vi "Convert64PinPGAToInputs.vi"(11 "64-Pin PGA":T2) -> (3 "Inputs":T1[](array[typedef]))   [LabVIEW 2012, in "Virtual-PGA.lvlib"]
uses:
  Virtual-PGA.lvlib
  Public/Controls/64PinPGAPattern.ctl
  Public/Controls/64PinPGAPads1-16.ctl
  Public/Controls/64PinPGAPad1-16.ctl
  Public/Controls/64PinPGAPads17-32.ctl
  Public/Controls/64PinPGAPad17-32.ctl
  Public/Controls/64PinPGAPads33-48.ctl
  Public/Controls/64PinPGAPad33-48.ctl
  Public/Controls/64PinPGAPads49-64.ctl
  Public/Controls/64PinPGAPad49-64.ctl
  Public/Controls/Input.ctl
panel:
  # "Name:"
  # "Inputs:"
  # "Description:"
  # "Y4:"
  # "Y3:"
  # "Y2:"
  # "Y1:"
  # "49"
  # "50"
  # "51"
  # "52"
  # "53"
  # "54"
  # "55"
  # "56"
  # "57"
  # "58"
  # "59"
  # "60"
  # "61"
  # "62"
  # "63"
  # "64"
  # "1"
  # "2"
  # "3"
  # "4"
  # "5"
  # "6"
  # "7"
  # "8"
  # "9"
  # "10"
  # "11"
  # "12"
  # "13"
  # "14"
  # "15"
  # "16"
  # "32"
  # "31"
  # "30"
  # "29"
  # "28"
  # "27"
  # "26"
  # "25"
  # "24"
  # "23"
  # "22"
  # "21"
  # "20"
  # "19"
  # "18"
  # "17"
  # "48"
  # "47"
  # "46"
  # "45"
  # "44"
  # "43"
  # "42"
  # "41"
  # "40"
  # "39"
  # "38"
  # "37"
  # "36"
  # "35"
  # "34"
  # "33"
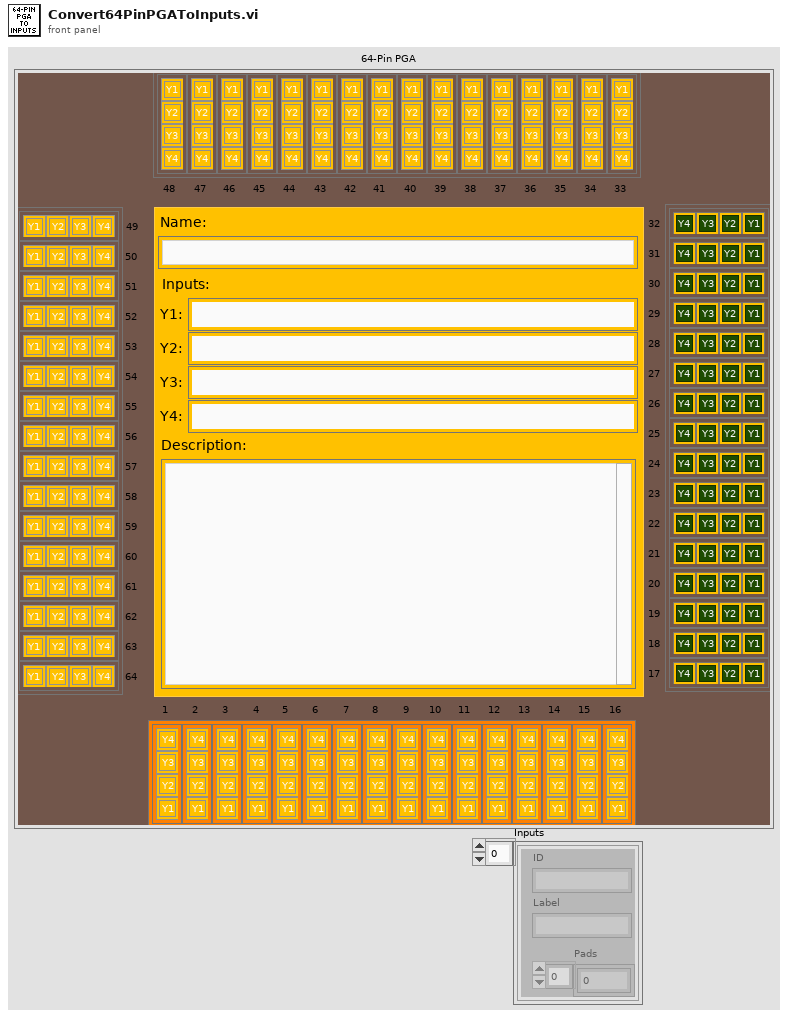
[diagram p1: front panel]
types:
  T1 = typedef "Virtual-PGA.lvlib/Input.ctl" = cluster{"ID":string, "Label":string, "Pads":u32[]}
  T2 = typedef "Virtual-PGA.lvlib/64PinPGAPattern.ctl" = cluster{"Name":string, "Description":string, "Y1 Label":string, "Y2 Label":string, "Y3 Label":string, "Y4 Label":string, "Pads 1-16":T3, "Pads 17-32":T5, "Pads 33-48":T7, "Pads 49-64":T9}
  T3 = typedef "Virtual-PGA.lvlib/64PinPGAPads1-16.ctl" = T4[]
  T4 = typedef "Virtual-PGA.lvlib/64PinPGAPad1-16.ctl" = cluster{"Y1":bool, "Y2":bool, "Y3":bool, "Y4":bool}
  T5 = typedef "Virtual-PGA.lvlib/64PinPGAPads17-32.ctl" = T6[]
  T6 = typedef "Virtual-PGA.lvlib/64PinPGAPad17-32.ctl" = cluster{"Y1":bool, "Y2":bool, "Y3":bool, "Y4":bool}
  T7 = typedef "Virtual-PGA.lvlib/64PinPGAPads33-48.ctl" = T8[]
  T8 = typedef "Virtual-PGA.lvlib/64PinPGAPad33-48.ctl" = cluster{"Y1":bool, "Y2":bool, "Y3":bool, "Y4":bool}
  T9 = typedef "Virtual-PGA.lvlib/64PinPGAPads49-64.ctl" = T10[]
  T10 = typedef "Virtual-PGA.lvlib/64PinPGAPad49-64.ctl" = cluster{"Y1":bool, "Y2":bool, "Y3":bool, "Y4":bool}
  T11 = cluster{"Y1":bool, "Y2":bool, "Y3":bool, "Y4":bool}[]
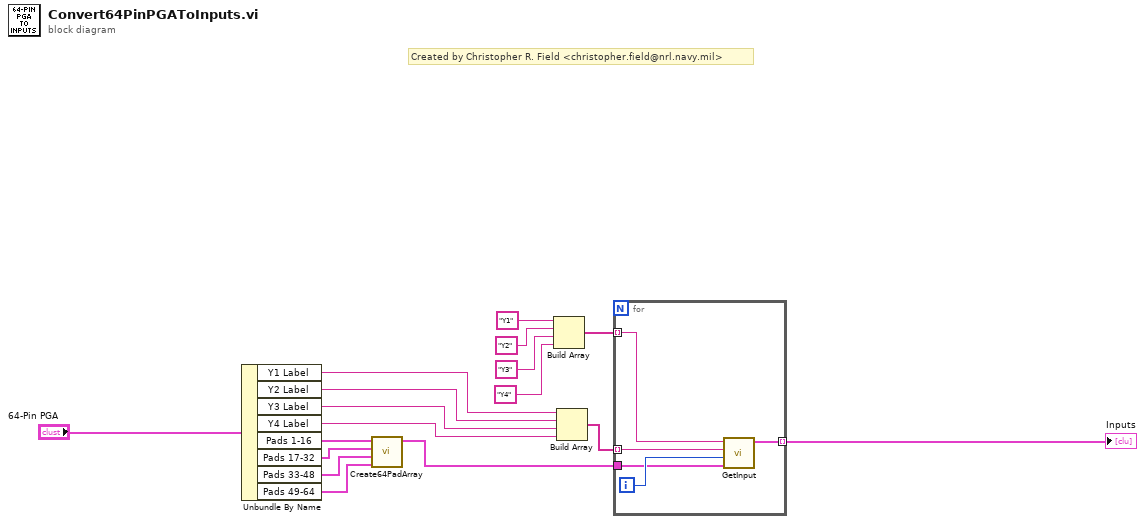
[diagram p0: block diagram]
diagram:
  # "Created by Christopher R. Field <christopher.field@nrl.navy.mil>"
  n1 = Unbundle By Name("64-Pin PGA") -> ("Y1 Label"=w6:string, "Y2 Label"=w5:string, "Y3 Label"=w4:string, "Y4 Label"=w3:string, "Pads 1-16"=w15:T3, "Pads 17-32"=w14:T5, "Pads 33-48"=w13:T7, "Pads 49-64"=w12:T9)
  n2 = call "Create64PadArray.vi"("Pads 49-64"=w12, "Pads 33-48"=w13, "Pads 17-32"=w14, "Pads 1-16"=w15) -> ("Pads 1-64"=w1:T11)  [unwired: 7 in]
  n3 = Build Array("Y1" ("Input ID"), "Y2" ("Input ID"), "Y3" ("Input ID"), "Y4" ("Input ID")) -> (w7:string[])
  n4 = Build Array(w6, w5, w4, w3) -> (w2:string[])
  n5 = for {
    tunnel: w7 -> [w21] mode=indexing
    tunnel: w2 -> [w22] mode=indexing
    tunnel: w1 -> [w19]
    tunnel: [w18] -> w16 mode=indexing
    i -> [w20]
    n6 = call "GetInput.vi"("Pads Array"=w19, "Input Index"=w20, "Input Label"=w22, "Input ID"=w21) -> ("Input"=w18:T1)  [unwired: 7 in]
  }
  "Inputs" <- w16
